vi "Encoder-Velocity_Conversion (SubVI).vi"(9 "delta  Encoder Count":i32, 11 "dt (uSec)":u32) -> (0 "Distance (ft)":dbl, 2 "Linear Velocity (ft/s)":dbl, 3 "Rotational Velocity (RPS)":dbl)   [LabVIEW 2015]
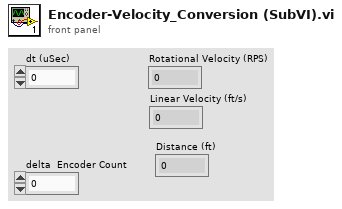
[diagram p1: front panel]
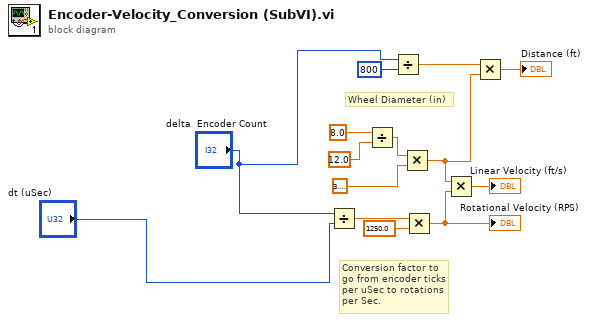
[diagram p0: block diagram]
diagram:
  # "Wheel Diameter (in)"
  # "Conversion factor to \ngo from encoder ticks \nper uSec to rotations\nper Sec."
  n1 = Divide(x="delta  Encoder Count", y="dt (uSec)") -> (x/y=w13:dbl)
  n2 = Divide(x=8.0, y=12.0) -> (x/y=w7:dbl)
  n3 = Divide(x="delta  Encoder Count", y=800) -> (x/y=w3:dbl)
  n4 = Multiply(x=w7, y=3.141592653589793) -> (x*y=w2:dbl)
  n5 = Multiply(x=w13, y=1250.0) -> (x*y=w11:dbl)
  "Rotational Velocity (RPS)" <- w11
  n6 = Multiply(x=w2, y=w11) -> (x*y=→"Linear Velocity (ft/s)":dbl)
  n7 = Multiply(x=w3, y=w2) -> (x*y=→"Distance (ft)":dbl)
